vi "PCE_TCP_READ.vi"(0 "ConnID IN":refnum<k5>, 7 "Timeout":u32, 11 "Error IN":errorcluster) -> (4 "ConnID OUT":refnum<k5>, 8 "Answer":string, 15 "Error OUT":errorcluster)   [LabVIEW 2010]
panel:
  out "String":string
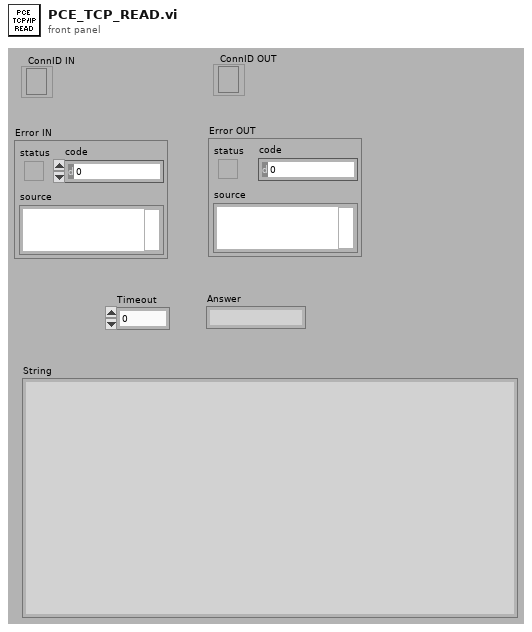
[diagram p1: front panel]
types:
  T1 = enum16{"Standard", "Buffered", "CRLF", "Immediate"}
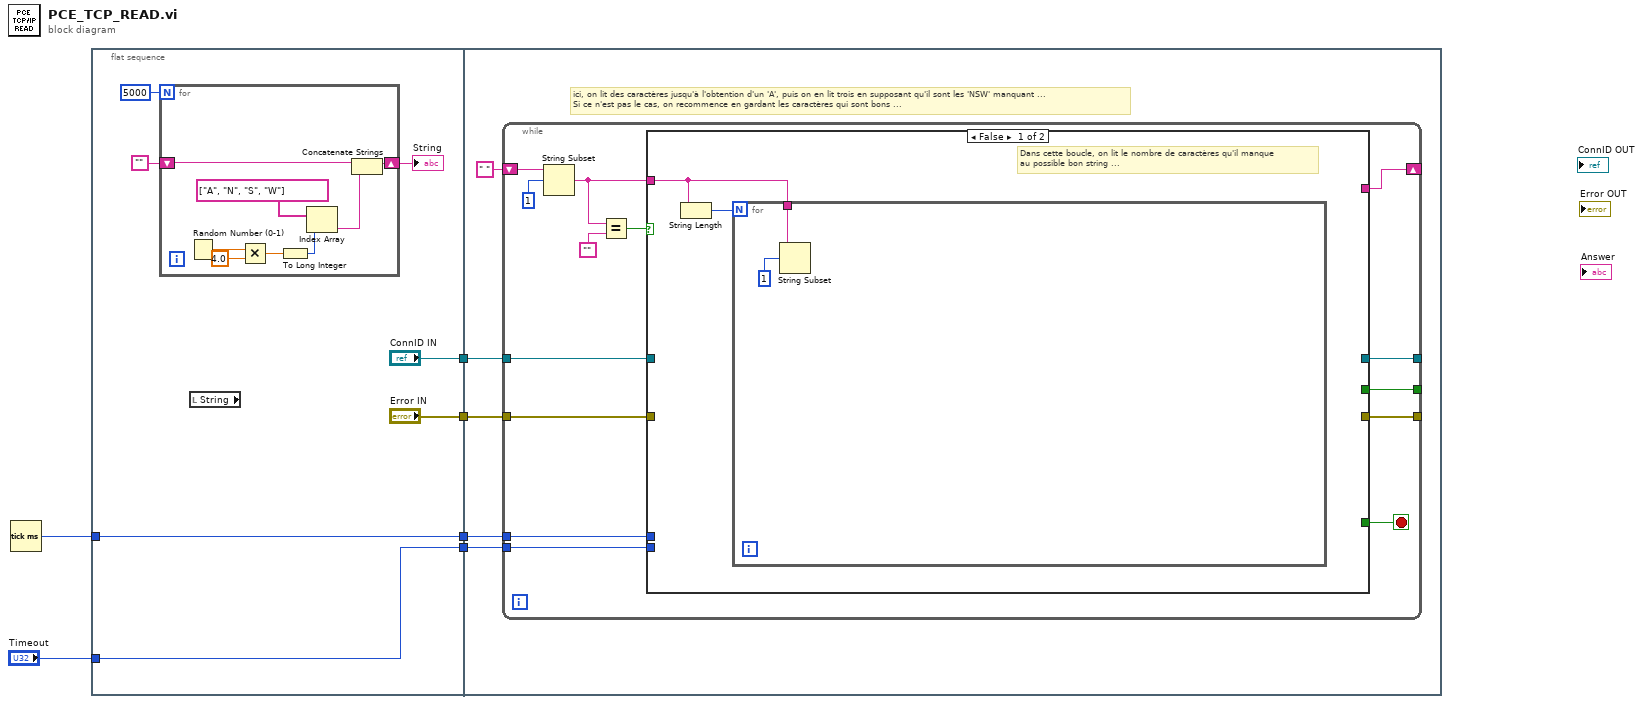
[diagram p0: block diagram]
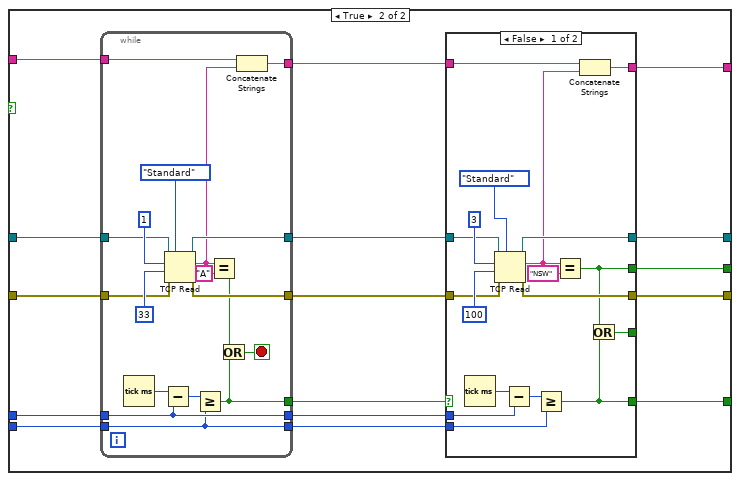
[diagram p2: hidden frame]
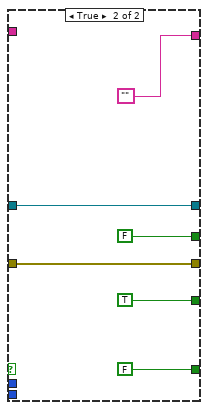
[diagram p3: hidden frame]
diagram:
  n1 = Tick Count (ms)() -> (millisecond timer value=w1:u32)
  n2 = flat-sequence {
    tunnel: "Timeout" -> [w11]
    tunnel: ["ConnID IN"] -> w5
    tunnel: ["Error IN"] -> w4
    tunnel: [w11] -> w3
    tunnel: [w10] -> w2
    tunnel: w1 -> [w10]
    tunnel: w5 -> [w26]
    tunnel: w4 -> [w25]
    tunnel: w3 -> [w24]
    tunnel: w2 -> [w23]
    frame #0 {
      n3 = for {
        N: 5000 -> [_]
        shift-right: [w16] -> w7
        shift-left: "" -> [w14]
        n4 = Random Number (0-1)() -> (number: 0 to 1=w20:dbl)
        n5 = Multiply(x=w20, y=4.0) -> (x*y=w19:dbl)
        n6 = To Long Integer(number=w19) -> (32bit integer=w18:i32)
        n7 = Index Array(array=string[] ["A", "N", "S", "W"], index=w18) -> (element=w15:string)
        n8 = Concatenate Strings(w14, w15) -> (w16:string)
      }
      "String" <- w7
      n9 = local read "String"() -> ()  [unwired: 1 out]
    }
    frame #1 {
      # "ici, on lit des caractères jusqu'à l'obtention d'un 'A', puis on en lit trois en supposant qu'il sont les 'NSW' manquant ...\nSi ce n'est pas le cas, on recommence en gardant les caractères qui sont bons ..."
      n10 = while {
        tunnel: w26 -> [w40]
        tunnel: w25 -> [w39]
        tunnel: w24 -> [w38]
        tunnel: w23 -> [w37]
        tunnel: [w35] -> _
        tunnel: [w34] -> _
        tunnel: [w33] -> _
        shift-right: [w32] -> _
        shift-left: " " -> [w29]
        stop <- w36 stop-if-true
        n11 = String Subset(string=w29, offset (0)=1 ("length (rest)")) -> (substring=w27:string)  [unwired: 1 in]
        n12 = Equal?(x=w27, y="") -> (x = y?=w31:bool)
        n13 = case shown="False" w31 {
          tunnel: w40 -> [_ w60]
          tunnel: w39 -> [_ w59]
          tunnel: w38 -> [_ w58]
          tunnel: w37 -> [_ w57]
          tunnel: [_ w56] -> w36
          tunnel: [_ w55] -> w35
          tunnel: [_ w54] -> w34
          tunnel: [_ w53] -> w33
          tunnel: w27 -> [w41 w52]
          tunnel: [_ w51] -> w32
          frame False {
            # "Dans cette boucle, on lit le nombre de caractères qu'il manque\nau possible bon string ..."
            n14 = String Length(string=w41) -> (length=w42:i32)
            n15 = for {
              N: w42 -> [_]
              tunnel: w41 -> [w43]
              n16 = String Subset(string=w43, offset (0)=1 ("length (rest)")) -> ()  [unwired: 1 in, 1 out]
            }
          }
          frame True {
            n17 = while {
              tunnel: w60 -> [w95]
              tunnel: w59 -> [w97]
              tunnel: w58 -> [w89]
              tunnel: w57 -> [w90]
              tunnel: [w96] -> w49
              tunnel: [w94] -> w50
              tunnel: [w92] -> w48
              tunnel: [w90] -> w47
              tunnel: [w89] -> w46
              tunnel: w52 -> [w88]
              tunnel: [w86] -> w45
              stop <- w93 stop-if-true
              n18 = Tick Count (ms)() -> (millisecond timer value=w101:u32)
              n19 = Subtract(x=w101, y=w90) -> (x-y=w99:u32)
              n20 = TCP Read(connection ID=w95, bytes to read=1, error in (no error)=w97, 7:T1."Standard" ("mode (standard)"), 9:33 ("timeout ms (25000)")) -> (connection ID out=w94:refnum<k5>, data out=w87:string, error out=w96:errorcluster)
              n21 = Greater Or Equal?(x=w99, y=w89) -> (x >= y?=w92:bool)
              n22 = Equal?(x=w87, y="A") -> (x = y?=w91:bool)
              n23 = Or(x=w91, y=w92) -> (x .or. y?=w93:bool)
              n24 = Concatenate Strings(w88, w87) -> (w86:string)
            }
            n25 = case shown="False" w48 {
              tunnel: w50 -> [w67 w81]
              tunnel: w49 -> [w69 w82]
              tunnel: [w70 FALSE] -> w56
              tunnel: w47 -> [w73 _]
              tunnel: w46 -> [w72 _]
              tunnel: [w71 TRUE] -> _
              tunnel: [w68 w82] -> w54
              tunnel: [w66 w81] -> w55
              tunnel: [w65 FALSE] -> w53
              tunnel: w45 -> [w64 _]
              tunnel: [w62 ""] -> w51
              frame False {
                n26 = Tick Count (ms)() -> (millisecond timer value=w74:u32)
                n27 = TCP Read(connection ID=w67, bytes to read=3, error in (no error)=w69, 7:T1."Standard" ("mode (standard)"), 9:100 ("timeout ms (25000)")) -> (connection ID out=w66:refnum<k5>, data out=w63:string, error out=w68:errorcluster)
                n28 = Subtract(x=w74, y=w73) -> (x-y=w75:u32)
                n29 = Greater Or Equal?(x=w75, y=w72) -> (x >= y?=w70:bool)
                n30 = Equal?(x=w63, y="NSW") -> (x = y?=w65:bool)
                n31 = Concatenate Strings(w64, w63) -> (w62:string)
                n32 = Or(x=w65, y=w70) -> (x .or. y?=w71:bool)
              }
              frame True {
              }
            }
          }
        }
      }
    }
  }
